vi "CheckIfNameIsCorrect.vi"(11 "Name":string) -> (3 "Correct?":bool)   [LabVIEW 2019]
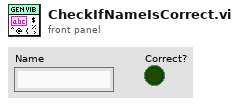
[diagram p1: front panel]
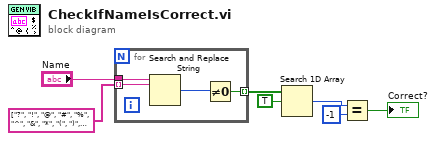
[diagram p0: block diagram]
diagram:
  n1 = for {
    tunnel: "Name" -> [w11]
    tunnel: string[] ["?", "!", "@", "#", "%", "^", "&", "*", "(", ")", "<", ">", ",", ".", ":", ";", "\"", "'", "{", "}", "[", "]", "+", "=", "~", "`"] -> [w10] mode=indexing
    tunnel: [w8] -> w3 mode=indexing
    n2 = Search and Replace String(input string=w11, search string=w10) -> (number of replacements=w9:i32)  [unwired: 6 in, 3 out]
    n3 = Not Equal To 0?(x=w9) -> (x != 0?=w8:bool)
  }
  n4 = Search 1D Array(1D array=w3, element=TRUE) -> (index of element=w6:i32)  [unwired: 1 in]
  n5 = Equal?(x=w6, y=-1) -> (x = y?=→"Correct?":bool)
